vi "SubVI RX MMSE.vi"(4 "b":cdb[](array[numeric]), 7 "A":cdb[][](array[numeric]) format="%0.2f") -> (0 "error code":i32, 2 "mean square error":dbl, 3 "x.estimate":cdb[](array[numeric]))   [LabVIEW 2015]
uses:
  <vilib>/Analysis/7linalg.llb/Complex Conjugate Transpose Matrix.vi
  <vilib>/Analysis/baseanly.llb/Complex A x B.vi
  <vilib>/Analysis/baseanly.llb/Complex A x Vector.vi
  <vilib>/Analysis/baseanly.llb/Complex Inverse Matrix.vi
  <vilib>/Analysis/NI_AALBase.lvlib
  <vilib>/Analysis/NI_AALPro.lvlib
panel:
  # "Linear MMSE estimator"
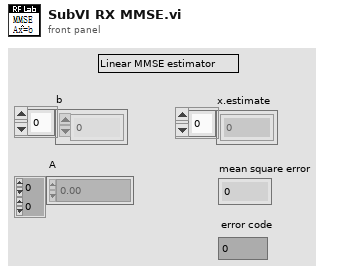
[diagram p1: front panel]
types:
  T1 = typedef "NI_Matrix.lvlib/ComplexMatrix.ctl" = cdb[][]
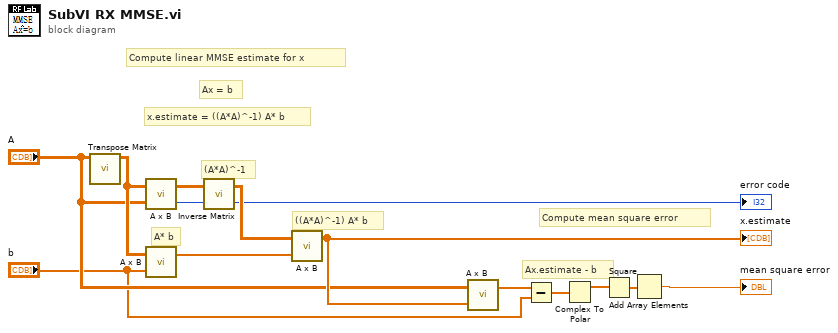
[diagram p0: block diagram]
diagram:
  # "Compute mean square error"
  # "Ax.estimate - b"
  # "x.estimate = ((A*A)^-1) A* b"
  # "Ax = b"
  # "Compute linear MMSE estimate for x"
  # "A* b"
  # "((A*A)^-1) A* b"
  # "(A*A)^-1"
  n1 = call-poly <vilib>:"Transpose Matrix.vi"("Input Matrix"="A") -> ("Matrix Conjugate Transpose"=w10:T1)  [unwired: 9 in, 1 out]
  n2 = call-poly <vilib>:"A x B.vi"("B"="A", "A"=w10) -> ("error"=w12:i32, "A x B"=w14:T1)
  n3 = call-poly <vilib>:"A x B.vi"("Vector"="b", "A"=w10) -> ("A x Vector"=w11:cdb[])  [unwired: 1 out]
  n4 = call-poly <vilib>:"Inverse Matrix.vi"("matrix type"=w12, "Input Matrix"=w14) -> ("error"=→"error code":i32, "Inverse Matrix"=w13:T1)
  n5 = call-poly <vilib>:"A x B.vi"("Vector"=w11, "A"=w13) -> ("A x Vector"=w5:cdb[])  [unwired: 1 out]
  "x.estimate" <- w5
  n6 = call-poly <vilib>:"A x B.vi"("Vector"=w5, "A"="A") -> ("A x Vector"=w7:cdb[])  [unwired: 1 out]
  n7 = Subtract(x=w7, y="b") -> (x-y=w8:cdb[])
  n8 = Complex To Polar(r * e^(i*theta)=w8) -> (r=w1:dbl[])  [unwired: 1 out]
  n9 = Square(x=w1) -> (x^2=w2:dbl[])
  n10 = Add Array Elements(numeric array=w2) -> (sum=→"mean square error":dbl)
